vi "01 Reading a voltage.vi"() -> ()   [LabVIEW 2019]
uses:
  <vilib>/Instr/_visa.llb/VISA Configure Serial Port (Instr).vi
panel:
  out "Connected":bool
  in  "stop":bool
  in  "Arduino code":string="/*\n  AnalogReadSerial\n\n  Reads an analog input on pin 0, prints the result to the Serial Monitor.\n  Graphical representation is available using Serial Plotter (Tools > Serial Plotter menu).\n  Attach the center pin of a potentiometer to pin A0, and the outside pins to +5V and ground.\n\n  This example code is in the public domain.\n\n  http://www.arduino.cc/en/Tutorial/AnalogReadSerial\n*/\n\n// the setup routine runs once when you press reset:\nvoid setup() {\n  // initialize serial communication at 9600 bits per second:\n  Serial.begin(9600);\n}\n\n// the loop routine runs over and over again forever:\nvoid loop() {\n  // read the input on analog pin 0:\n  int sensorValue = analogRead(A0);\n  // print out the value you read:\n  Serial.println(sensorValue);\n  delay(1);        // delay in between reads for stability\n}"
  in  "MicroPython Port":refnum<visa-resource-name>
  out "Gauge":i32(knob) scale=0.0..1000.0
  # "Download and run the MicroPython code below\n\nSelect the Arduino port below\n\nHit the Run arrow and see the Gauge change to the value of the sensor (read over serial)"
  # "Hit Cmd E to see the diagram (code)"
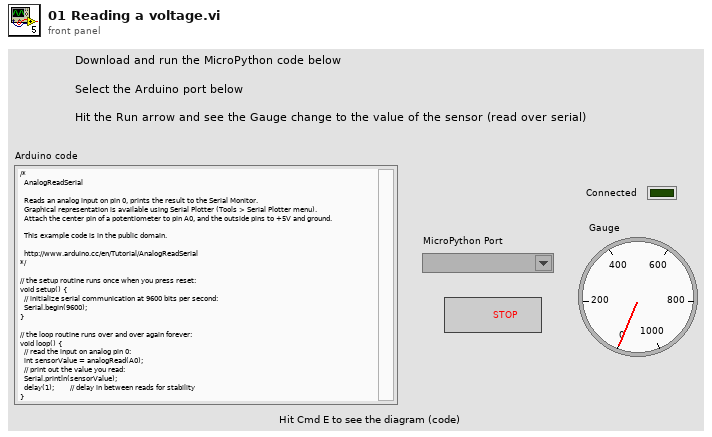
[diagram p1: front panel]
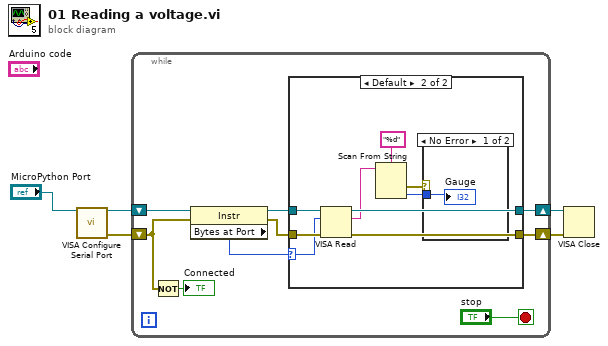
[diagram p0: block diagram]
diagram:
  n1 = call-poly "VISA Configure Serial Port"("VISA resource name"="MicroPython Port") -> ("VISA resource name out"=w4:refnum<visa-resource-name>, "error out"=w3:errorcluster)  [unwired: 13 in]
  n2 = while {
    shift-right: [w10] -> w1
    shift-left: w4 -> [w14]
    shift-right: [w11] -> w2
    shift-left: w3 -> [w7]
    stop <- "stop" stop-if-true
    n3 = Not(x=w7) -> (.not. x?=→"Connected":bool)
    n4 = property class="Instr"(reference=w14, error in=w7) -> (reference out=w13:refnum<visa-resource-name>, error out=w12:errorcluster, "Bytes at Port"=w8:u32)
    n5 = case shown="Default" w8 {
      selector: w8 -> [_ w21]
      tunnel: w13 -> [w16 w25]
      tunnel: w12 -> [w15 w24]
      tunnel: [w15 w23] -> w11
      tunnel: [w16 w22] -> w10
      frame 0 {
      }
      frame Default {
        n6 = VISA Read(VISA resource name=w25, byte count=w21, error in (no error)=w24) -> (VISA resource name out=w22:refnum<visa-resource-name>, read buffer=w19:string, error out=w23:errorcluster)  [unwired: 1 out]
        n7 = Scan From String(format string="%d", input string=w19) -> (error out=w18:errorcluster, output 1=w17:i32)  [unwired: 3 in, 2 out]
        n8 = case shown="No Error" w18 {
          tunnel: w17 -> [w26 _]
          frame No Error {
            "Gauge" <- w26
          }
          frame Error {
          }
        }
      }
    }
  }
  n9 = VISA Close(VISA resource name=w1, error in (no error)=w2) -> ()  [unwired: 1 out]
